vi "Launch RP Tester.vi"   [LabVIEW 2015]
uses:
  Red Pitaya Tester/Red Pitaya Tester.lvclass
  <vilib>/ActorFramework/Actor/Actor.lvclass
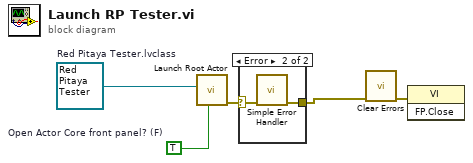
[diagram p0: block diagram]
diagram:
  w1 = TRUE  # Open Actor Core front panel? (F)
  w4 = refnum<class "Red Pitaya Tester.lvclass"> refnum  # Red Pitaya Tester.lvclass
  n1 = call <vilib>:"Launch Root Actor.vi"("Open Actor Core front panel? (F)"=w1, "Actor"=w4) -> ("error out"=w3:errorcluster)  [unwired: 8 in, 1 out]
  n2 = case shown="Error" w3 {
    selector: w3 -> [w6 w8]
    tunnel: [w6 w7] -> w2
    frame No Error {
    }
    frame Error {
      n3 = call <vilib>:"Simple Error Handler.vi"("error in (no error)"=w8) -> ("error out"=w7:errorcluster)  [unwired: 4 in, 4 out]
    }
  }
  n4 = call <vilib>:"Clear Errors.vi"("error in (no error)"=w2) -> ("error out"=w5:errorcluster)  [unwired: 5 in, 1 out]
  n5 = invoke class="VI" method="FP.Close"(error in=w5) -> ()  [unwired: 2 in, 3 out]
